vi "GetHWI.vi"(8 "error in (no error)":errorcluster, 11 "Pulseblaster in":refnum<class "Pulseblaster.lvclass">) -> (0 "error out":errorcluster, 2 "Hardware Image":T1, 3 "Pulseblaster out":refnum<class "Pulseblaster.lvclass">)   [LabVIEW 2013, in "Pulseblaster.lvclass"]
uses:
  Pulseblaster.lvclass
  Pulseblaster.lvclass/Pulseblaster.ctl
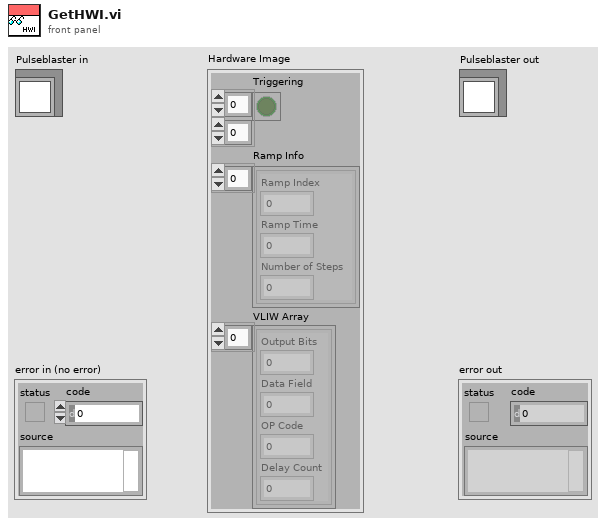
[diagram p1: front panel]
types:
  T1 = cluster{"Triggering":bool[][], "Ramp Info":cluster{"Ramp Index":i32, "Ramp Time":dbl, "Number of Steps":i32}[], "VLIW Array":cluster{"Output Bits":u32, "Data Field":u32, "OP Code":u8, "Delay Count":u64}[]}
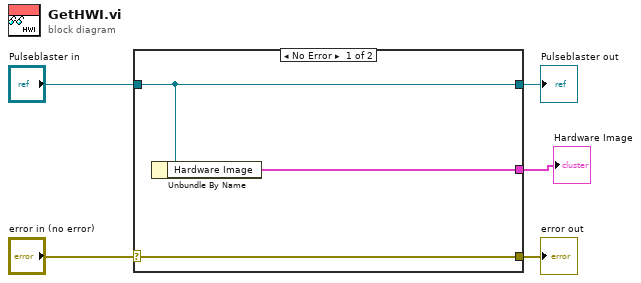
[diagram p0: block diagram]
diagram:
  n1 = case shown="No Error" "error in (no error)" {
    selector: "error in (no error)" -> [w8 w9]
    tunnel: [w8 w9] -> w4
    tunnel: [w7 w10] -> w2
    tunnel: "Pulseblaster in" -> [w7 w10]
    tunnel: [w6 _] -> w1
    frame No Error {
      n2 = Unbundle By Name(w7) -> ("Hardware Image"=w6:T1)
    }
    frame Error {
    }
  }
  "error out" <- w4
  "Pulseblaster out" <- w2
  "Hardware Image" <- w1
